vi "get files list.vi"(8 "error in":errorcluster, 11 "Cluster in":T1={"This VI Ref"=refnum, "Test VI"=refnum, "Q Ref"=refnum, "UE"=refnum, "Data"=variant, "Timeout"=-1, "Path List[]"=[], "Status"="", "Counter"=0, "Config"={"Source Path"=path "", "Dest Path"=path "", "Log Path"=path "", "Move?"=FALSE, "Log?"=FALSE, "Scanners"=[], "Excude Folders"=[], "Jpg?"=FALSE, "Default path"=path "", "Extended?"=FALSE, "Mode"=enum."Move", "Temp"=FALSE}, "Total"=0, "Config Path"=path "", "exif info"={"Make"="Canon\u0000", "Model"="Canon PowerShot A495\u0000", "Orientation"=0, "Date"=timestamp(0 s since 1904-01-01), "Width"=0, "Height"=0, "Square?"=FALSE, "File Name"="Canon\u0000", "Extension"="Canon\u0000", "Valid?"=FALSE, "Path"=path "", "size"=0, "No Ext?"=FALSE, "prefix?"=FALSE, "Tag"="", "Name Type"=enum."Event Sufix", "Projection Type"="Canon\u0000"}, "app operation"=enum."Start", "Log Ref"=refnum, "Start Time"=0.0, "Pause Time"=0.0, "Argument?"=FALSE, "Argument path"=path "", "Identical"=FALSE, "File.lvclass"=refnum}) -> (0 "error out":errorcluster, 3 "Cluster out":T1={"This VI Ref"=refnum, "Test VI"=refnum, "Q Ref"=refnum, "UE"=refnum, "Data"=variant, "Timeout"=-1, "Path List[]"=[], "Status"="", "Counter"=0, "Config"={"Source Path"=path "", "Dest Path"=path "", "Log Path"=path "", "Move?"=FALSE, "Log?"=FALSE, "Scanners"=[], "Excude Folders"=[], "Jpg?"=FALSE, "Default path"=path "", "Extended?"=FALSE, "Mode"=enum."Move", "Temp"=FALSE}, "Total"=0, "Config Path"=path "", "exif info"={"Make"="Canon\u0000", "Model"="Canon PowerShot A495\u0000", "Orientation"=0, "Date"=timestamp(0 s since 1904-01-01), "Width"=0, "Height"=0, "Square?"=FALSE, "File Name"="Canon\u0000", "Extension"="Canon\u0000", "Valid?"=FALSE, "Path"=path "", "size"=0, "No Ext?"=FALSE, "prefix?"=FALSE, "Tag"="", "Name Type"=enum."Event Sufix", "Projection Type"="Canon\u0000"}, "app operation"=enum."Start", "Log Ref"=refnum, "Start Time"=0.0, "Pause Time"=0.0, "Argument?"=FALSE, "Argument path"=path "", "Identical"=FALSE, "File.lvclass"=refnum})   [LabVIEW 2023, in "User Interface.lvlib"]
uses:
  User Interface.lvlib
  Controls/main consumer cluster.ctl
  File Classes/File/File.lvclass
  Controls/configuration cluster.ctl
  File Classes/Controls/exif data cluster.ctl
  File Classes/Controls/rename type enum.ctl
  Controls/app operation state enum.ctl
  File Classes/File Classes.lvlib
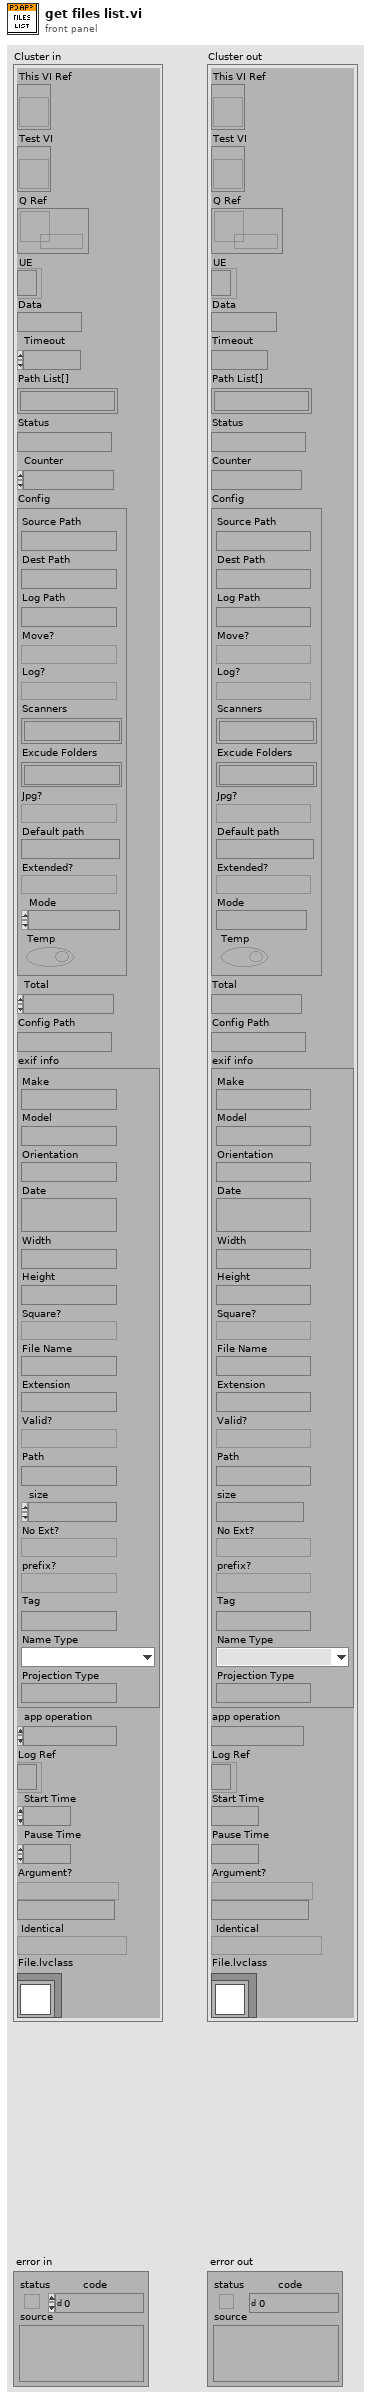
[diagram p1: front panel]
types:
  T1 = typedef "User Interface.lvlib/main consumer cluster.ctl" = cluster{"This VI Ref":refnum<vi>, "Test VI":refnum<vi>, "Q Ref":refnum<queue>, "UE":refnum<event-registration>, "Data":variant, "Timeout":i32, "Path List[]":path[], "Status":string, "Counter":i32, "Config":T2, "Total":i32, "Config Path":path, "exif info":T3, "app operation":T5, "Log Ref":refnum<file>, "Start Time":dbl, "Pause Time":dbl, "Argument?":bool, "Argument path":path, "Identical":bool, "File.lvclass":refnum<class "File.lvclass">}
  T2 = typedef "User Interface.lvlib/configuration cluster.ctl" = cluster{"Source Path":path, "Dest Path":path, "Log Path":path, "Move?":bool, "Log?":bool, "Scanners":string[], "Excude Folders":string[], "Jpg?":bool, "Default path":path, "Extended?":bool, "Mode":enum16{"Copy (Default)", "Move", "Rename"}, "Temp":bool}
  T3 = typedef "File Classes.lvlib/exif data cluster.ctl" = cluster{"Make":string, "Model":string, "Orientation":u16, "Date":timestamp, "Width":u16, "Height":u16, "Square?":bool, "File Name":string, "Extension":string, "Valid?":bool, "Path":path, "size":i64, "No Ext?":bool, "prefix?":bool, "Tag":string, "Name Type":T4, "Projection Type":string}
  T4 = typedef "File Classes.lvlib/rename type enum.ctl" = enum16{"Date & Time (Default)", "Model Sufix", "Event Sufix", "Model & Event Sufix"}
  T5 = typedef "User Interface.lvlib/app operation state enum.ctl" = enum16{"Start", "Stop", "Pause", "Resume"}
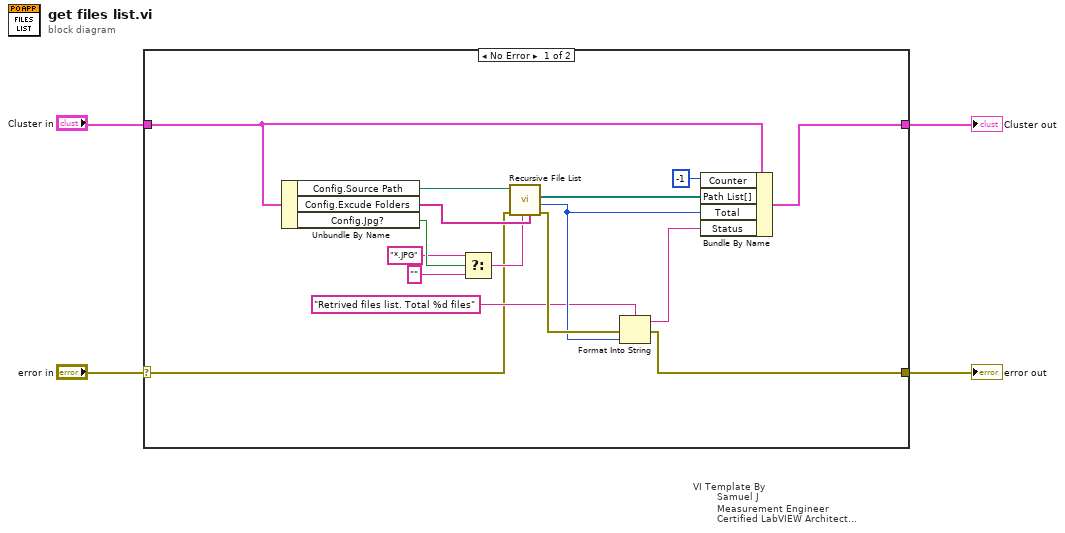
[diagram p0: block diagram]
diagram:
  n1 = case "VI Template By\n        Samuel J\n        Measurement Engineer\n        Certified LabVIEW Architect\n        Vestas Technology R&D Chennai" shown="No Error" "error in" {
    selector: "error in" -> [w8 w22]
    tunnel: [w7 w22] -> w3
    tunnel: [w6 w21] -> w2
    tunnel: "Cluster in" -> [w5 w21]
    frame No Error {
      n2 = Unbundle By Name(w5) -> ("Config.Source Path"=w20:path, "Config.Excude Folders"=w14:string[], "Config.Jpg?"=w13:bool)
      n3 = Select(t="*.JPG" ("format string"), s=w13, f="") -> (s? t:f=w10:string)
      n4 = call <vilib>:"Recursive File List.vi"("Folders to Exclude"=w14, "pattern"=w10, "error in (no error)"=w8, "Folder Path"=w20) -> ("error out"=w18:errorcluster, "Number of Files"=w16:i32, "All Files in Dir"=w19:path[])  [unwired: 3 in, 2 out]
      n5 = Format Into String(format string="Retrived files list. Total %d files", error in=w18, w16) -> (resulting string=w17:string, error out=w7:errorcluster)  [unwired: 1 in]
      n6 = Bundle By Name(cluster=w5, "Counter"=-1, "Path List[]"=w19, "Total"=w16, "Status"=w17) -> (w6:T1)
    }
    frame Error {
    }
  }
  "error out" <- w3
  "Cluster out" <- w2
